vi "Calculate Plot Range.vi"(8 "error in (no error)":errorcluster, 10 "2D Compass Datatype.lvclass in":refnum<class "2D Compass Datatype.lvclass">, 11 "Plot Representation In":T1) -> (0 "error out":errorcluster, 2 "2D Compass Datatype.lvclass out":refnum<class "2D Compass Datatype.lvclass">, 3 "Plot Representation Out":T1)   [LabVIEW 2017, in "2D Compass Datatype.lvclass"]
uses:
  <vilib>/Math Plots/2D Math Plots/2D Compass/2D Compass Datatype/2D Compass Datatype.lvclass
  <vilib>/Math Plots/2D Math Plots/2D Plot/2D Plot/Typedef/Plot Representation.ctl
  <vilib>/Math Plots/2D Math Plots/2D Plot/2D Plot/Typedef/Range Cluster.ctl
  <vilib>/Math Plots/2D Math Plots/2D Plot/2D Plot/2D Plot.lvclass
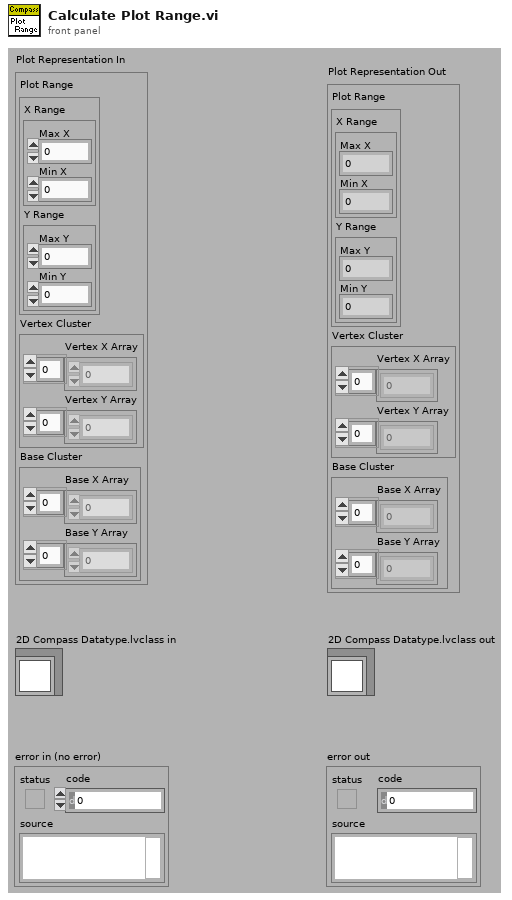
[diagram p1: front panel]
types:
  T1 = typedef "2D Plot.lvclass/Plot Representation.ctl" = cluster{"Plot Range":T2, "Vertex Cluster":cluster{"Vertex X Array":dbl[], "Vertex Y Array":dbl[]}, "Base Cluster":cluster{"Base X Array":dbl[], "Base Y Array":dbl[]}}
  T2 = typedef "2D Plot.lvclass/Range Cluster.ctl" = cluster{"X Range":cluster{"Max X":dbl, "Min X":dbl}, "Y Range":cluster{"Max Y":dbl, "Min Y":dbl}}
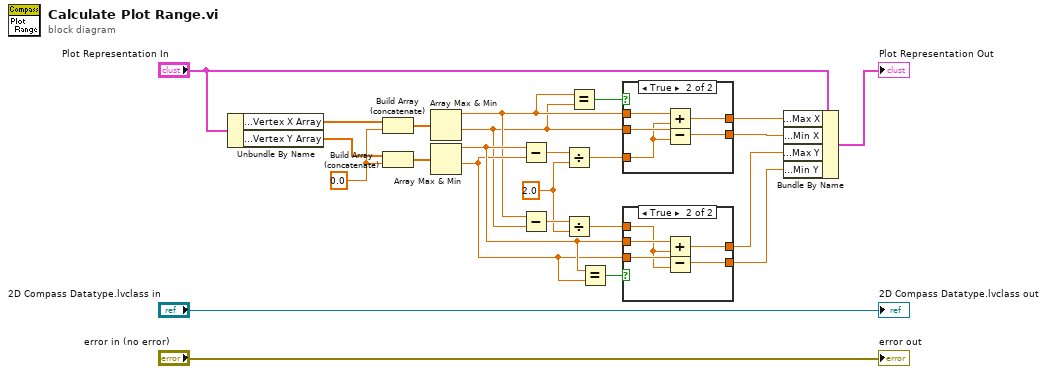
[diagram p0: block diagram]
diagram:
  w1 = 2.0 ("y")
  w16 = 0.0
  n1 = Unbundle By Name("Plot Representation In") -> ("Vertex Cluster.Vertex X Array"=w20:dbl[], "Vertex Cluster.Vertex Y Array"=w19:dbl[])
  n2 = Build Array (concatenate)(w20, w16) -> (w18:dbl[])
  n3 = Build Array (concatenate)(w19, w16) -> (w17:dbl[])
  n4 = Array Max & Min(array=w18) -> (max value=w4:dbl, min value=w3:dbl)  [unwired: 2 out]
  n5 = Array Max & Min(array=w17) -> (max value=w8:dbl, min value=w7:dbl)  [unwired: 2 out]
  n6 = Subtract(x=w8, y=w7) -> (x-y=w12:dbl)
  n7 = Subtract(x=w4, y=w3) -> (x-y=w5:dbl)
  n8 = Divide(x=w12, y=w1) -> (x/y=w11:dbl)
  n9 = Divide(x=w5, y=w1) -> (x/y=w2:dbl)
  n10 = Equal?(x=w4, y=w3) -> (x = y?=w15:bool)
  n11 = Equal?(x=w8, y=w7) -> (x = y?=w6:bool)
  n12 = case shown="True" w15 {
    tunnel: w4 -> [w26 w31]
    tunnel: w3 -> [w25 w29]
    tunnel: [w26 w30] -> w14
    tunnel: [w25 w28] -> w13
    tunnel: w11 -> [_ w27]
    frame False {
    }
    frame True {
      n13 = Add(x=w31, y=w27) -> (x+y=w30:dbl)
      n14 = Subtract(x=w29, y=w27) -> (x-y=w28:dbl)
    }
  }
  n15 = case shown="True" w6 {
    tunnel: w8 -> [w33 w38]
    tunnel: w7 -> [w32 w36]
    tunnel: [w33 w37] -> w10
    tunnel: [w32 w35] -> w9
    tunnel: w2 -> [_ w34]
    frame False {
    }
    frame True {
      n16 = Add(x=w38, y=w34) -> (x+y=w37:dbl)
      n17 = Subtract(x=w36, y=w34) -> (x-y=w35:dbl)
    }
  }
  n18 = Bundle By Name(cluster="Plot Representation In", "Plot Range.X Range.Max X"=w14, "Plot Range.X Range.Min X"=w13, "Plot Range.Y Range.Max Y"=w10, "Plot Range.Y Range.Min Y"=w9) -> (→"Plot Representation Out":T1)
  "2D Compass Datatype.lvclass out" <- "2D Compass Datatype.lvclass in"
  "error out" <- "error in (no error)"
